vi "report timing.vi"(9 "status reporting tags":T3={"late? index (bool)"=0, "late count index (U32)"=0, "dt (ns) index (U64)"=0, "execution time (ns) index (U64)"=-1}, 10 "time data in":T1, 11 "engine tag bus":T2) -> (2 "time data out":T1, 3 "engine data out":T2)   [LabVIEW 2013, in "main engine.lvlib"]
doc: "This VI writes to any of the timing or error tags that have been configured based on the results of this iteration of the loop."
uses:
  main engine.lvlib
  status reporting data.ctl
  <vilib>/NI/Tag Bus/table/data table.ctl
  time information.ctl
  <vilib>/NI/Tag Bus/table/data polymorphs/write one/write Boolean.vi
  <vilib>/NI/Tag Bus/table/data polymorphs/write one/write U32.vi
  <vilib>/NI/Tag Bus/table/data polymorphs/write one/write U64.vi
  <vilib>/NI/Tag Bus/table/data table.lvlib
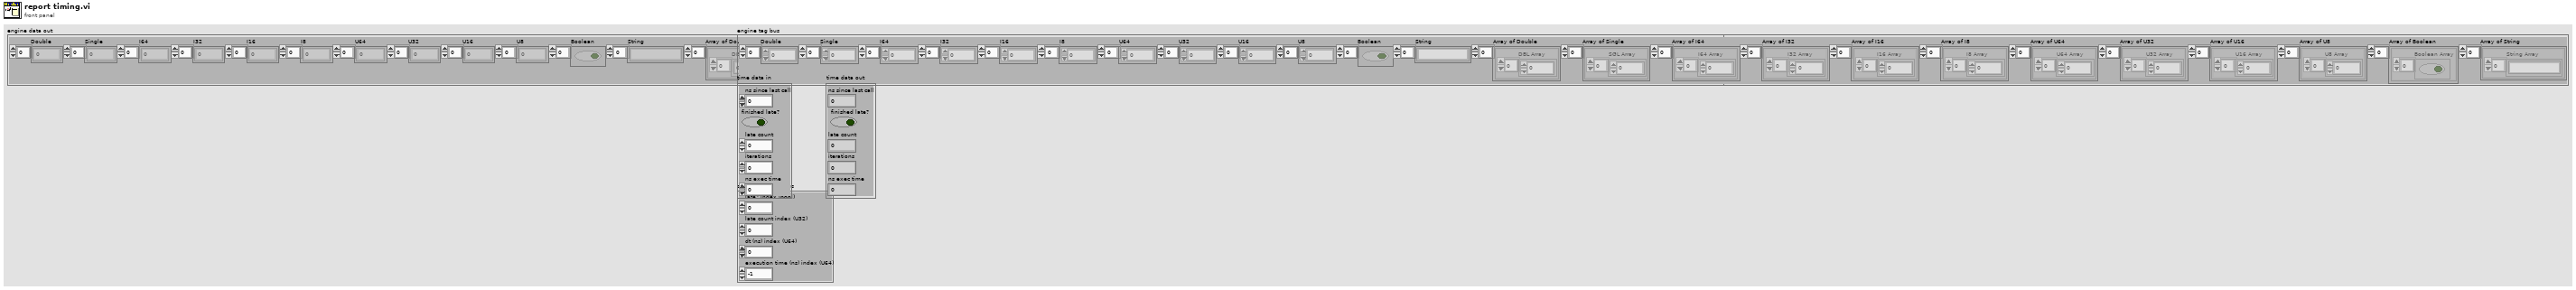
[diagram p1: front panel]
types:
  T1 = typedef "main engine.lvlib/time information.ctl" = cluster{"ns since last call":u64, "finished late?":bool, "late count":u32, "iterations":u64, "ns exec time":u64}
  T2 = typedef "tag bus.lvlib/data table.lvlib/data table.ctl" = cluster{"Double":dbl[], "Single":sgl[], "I64":i64[], "I32":i32[], "I16":i16[], "I8":i8[], "U64":u64[], "U32":u32[], "U16":u16[], "U8":u8[], "Boolean":bool[], "String":string[], "Array of Double":cluster{"DBL Array":dbl[]}[], "Array of Single":cluster{"SGL Array":sgl[]}[], "Array of I64":cluster{"I64 Array":i64[]}[], "Array of I32":cluster{"I32 Array":i32[]}[], "Array of I16":cluster{"I16 Array":i16[]}[], "Array of I8":cluster{"I8 Array":i8[]}[], "Array of U64":cluster{"U64 Array":u64[]}[], "Array of U32":cluster{"U32 Array":u32[]}[], "Array of U16":cluster{"U16 Array":u16[]}[], "Array of U8":cluster{"U8 Array":u8[]}[], "Array of Boolean":cluster{"Boolean Array":bool[]}[], "Array of String":cluster{"String Array":string[]}[]}
  T3 = typedef "main engine.lvlib/status reporting data.ctl" = cluster{"late? index (bool)":i32, "late count index (U32)":i32, "dt (ns) index (U64)":i32, "execution time (ns) index (U64)":i32}
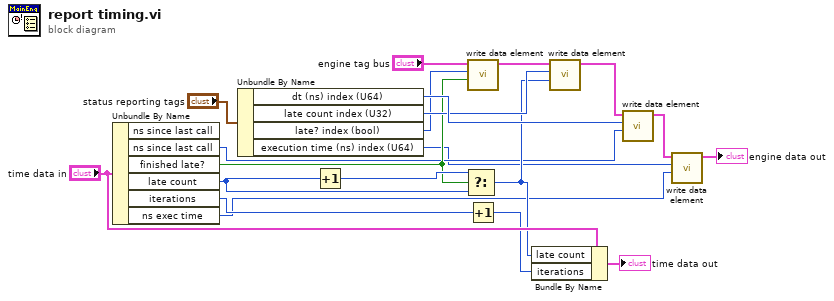
[diagram p0: block diagram]
diagram:
  n1 = Unbundle By Name("time data in") -> ("ns since last call"=w5:u64, "finished late?"=w6:bool, "late count"=w7:u32, "iterations"=w8:u64, "ns exec time"=w2:u64)  [unwired: 1 out]
  n2 = Unbundle By Name("status reporting tags") -> ("dt (ns) index (U64)"=w20:i32, "late count index (U32)"=w19:i32, "late? index (bool)"=w18:i32, "execution time (ns) index (U64)"=w1:i32)
  n3 = Increment(x=w7) -> (x+1=w13:u32)
  n4 = Select(t=w13, s=w6, f=w7) -> (s? t:f=w10:u32)
  n5 = call-poly <vilib>:"write data element.vi"("value"=w6, "index"=w18, "data table in"="engine tag bus") -> ("data table out"=w15:T2)  [unwired: 8 in]
  n6 = Increment(x=w8) -> (x+1=w9:u64)
  n7 = Bundle By Name(cluster="time data in", "late count"=w10, "iterations"=w9) -> (→"time data out":T1)
  n8 = call-poly <vilib>:"write data element.vi"("value"=w10, "index"=w19, "data table in"=w15) -> ("data table out"=w14:T2)  [unwired: 8 in]
  n9 = call-poly <vilib>:"write data element.vi"("value"=w5, "index"=w20, "data table in"=w14) -> ("data table out"=w4:T2)  [unwired: 8 in]
  n10 = call-poly <vilib>:"write data element.vi"("value"=w2, "index"=w1, "data table in"=w4) -> ("data table out"=→"engine data out":T2)  [unwired: 8 in]
